vi "Write Dialog Listbox values.vi"(9 "Label.Text":string="Phase Shift, deg", 10 "Values":dbl[](array[numeric]), 11 "module ref":refnum<vi>) -> (1 "Names, len":i32)   [LabVIEW 2017]
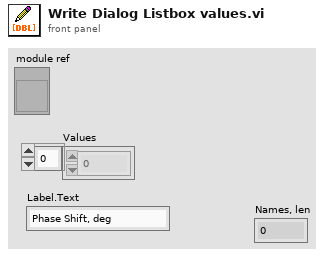
[diagram p1: front panel]
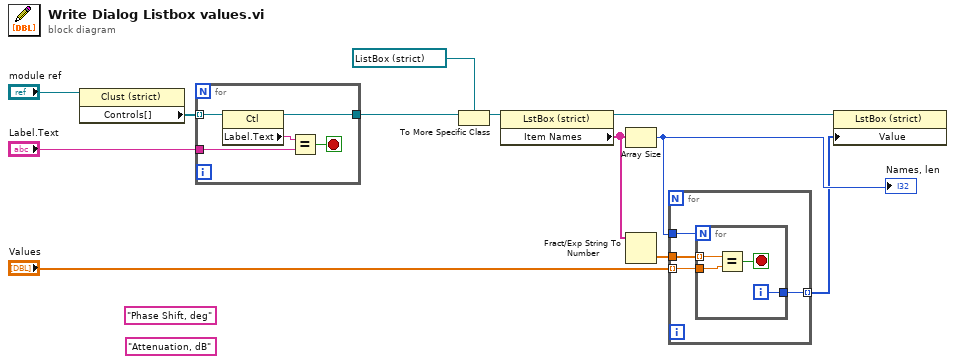
[diagram p0: block diagram]
diagram:
  (unwired) "Phase Shift, deg" ("Label.Text")
  (unwired) "Attenuation, dB" ("Label.Text")
  n1 = property class="Clust (strict)"(reference="module ref") -> ("Controls[]"=w12:refnum<vi>[])  [unwired: 1 in, 2 out]
  n2 = for {
    tunnel: w12 -> [w17] mode=indexing
    tunnel: "Label.Text" -> [w16]
    tunnel: [w13] -> w10
    stop <- w14 stop-if-true
    n3 = property class="Ctl"(reference=w17) -> (reference out=w13:refnum<vi>, "Label.Text"=w15:string)  [unwired: 1 in, 1 out]
    n4 = Equal?(x=w15, y=w16) -> (x = y?=w14:bool)
  }
  n5 = To More Specific Class(target class=refnum<vi> refnum ("Phase Shift, deg"), reference=w10) -> (specific class reference=w8:refnum<vi>)  [unwired: 1 in, 1 out]
  n6 = property class="LstBox (strict)"(reference=w8) -> (reference out=w2:refnum<vi>, "Item Names"=w4:string[])  [unwired: 1 in, 1 out]
  n7 = Array Size(array=w4) -> (size(s)=w5:i32)
  "Names, len" <- w5
  n8 = Fract/Exp String To Number(string=w4) -> (number=w3:dbl[])  [unwired: 3 in, 1 out]
  n9 = for {
    tunnel: "Values" -> [w19] mode=indexing
    tunnel: w3 -> [w21]
    tunnel: w5 -> [w20]
    tunnel: [w18] -> w1 mode=indexing
    n10 = for {
      N: w20 -> [_]
      tunnel: w21 -> [w24] mode=indexing
      tunnel: w19 -> [w23]
      tunnel: [w22] -> w18
      i -> [w22]
      stop <- w25 stop-if-true
      n11 = Equal?(x=w24, y=w23) -> (x = y?=w25:bool)
    }
  }
  n12 = property class="LstBox (strict)"(reference=w2, "Value"=w1) -> ()  [unwired: 1 in, 2 out]
